vi "File Operation.vi"(8 "error in (no error)":errorcluster, 10 "Enum":T2, 11 "Cluster":T1) -> (0 "error out":errorcluster, 3 "Array":T1[][](array[typedef]))   [LabVIEW 2020]
uses:
  Controller/Product controller.ctl
  Controller/File Operation Controller.ctl
  <vilib>/Utility/config.llb/Read Key (String).vi
  <vilib>/Utility/config.llb/Read Key (I32).vi
  <vilib>/Utility/config.llb/Write Key (String).vi
  <vilib>/Utility/config.llb/NI_LVConfig.lvlib
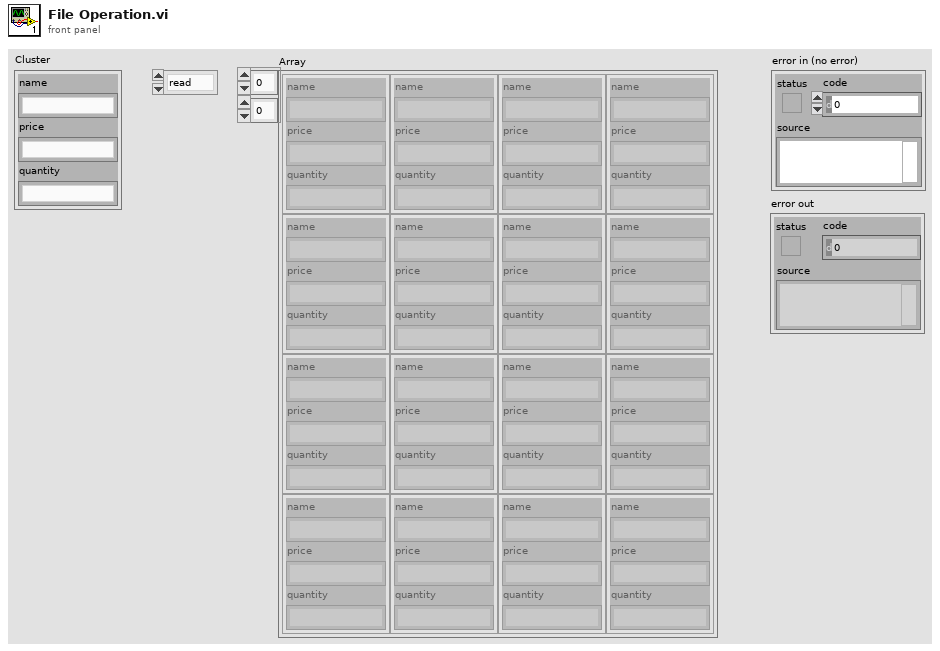
[diagram p1: front panel]
types:
  T1 = typedef "Product controller.ctl" = cluster{"name":string, "price":string, "quantity ":string}
  T2 = typedef "File Operation Controller.ctl" = enum16{"read", "write"}
  T3 = typedef "NI_LVConfig.lvlib/Config Data RefNum.ctl" = refnum<k1>
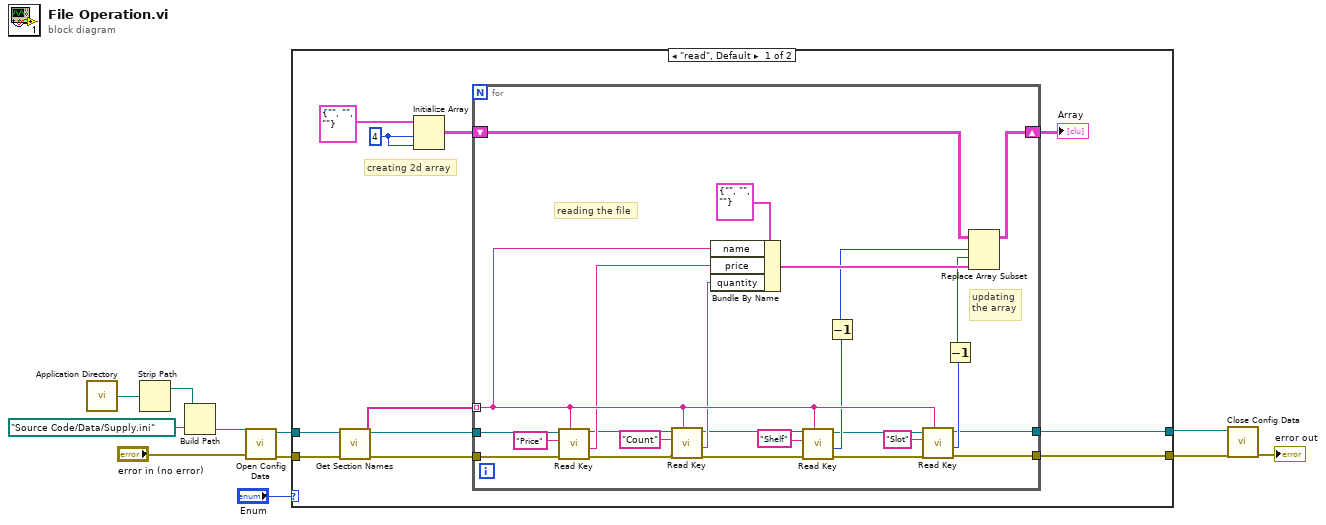
[diagram p0: block diagram]
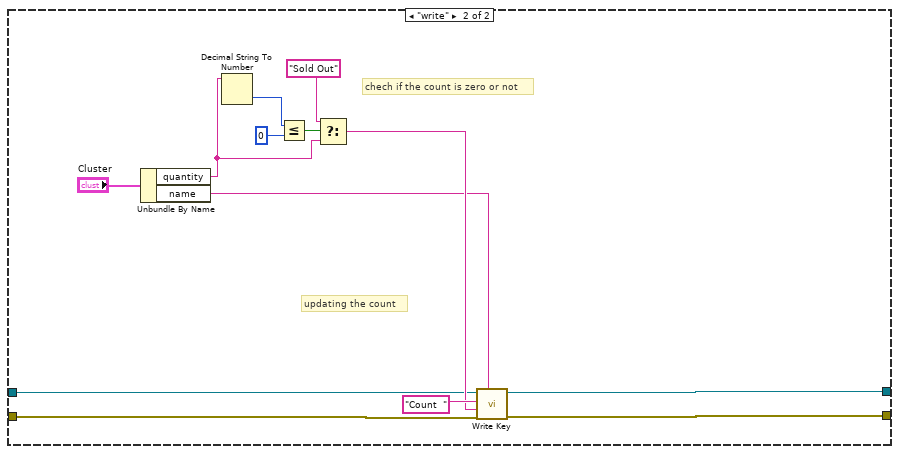
[diagram p2: hidden frame]
diagram:
  n1 = call <vilib>:"Application Directory.vi"() -> ("Application Directory"=w2:path)
  n2 = Strip Path(path=w2) -> (stripped path=w4:path)  [unwired: 1 out]
  n3 = Build Path(base path=w4, name or relative path=path "Source Code/Data/Supply.ini") -> (appended path=w1:path)
  n4 = call <vilib>:"Open Config Data.vi"("error in (no error)"="error in (no error)", "configuration file path"=w1) -> ("error out"=w10:errorcluster, "refnum"=w9:T3)  [unwired: 7 in, 1 out]
  n5 = case shown="\"read\", Default" "Enum" {
    tunnel: w10 -> [w21 w50]
    tunnel: w9 -> [w22 w51]
    tunnel: [w13 w57] -> w7
    tunnel: [w14 w58] -> w8
    frame "read", Default {
      w18 = 4 ("dimension size")
      # "creating 2d array"
      n6 = call <vilib>:"Get Section Names.vi"("error in (no error)"=w21, "refnum"=w22) -> ("error out"=w15:errorcluster, "section names"=w20:string[], "refnum out"=w12:T3)  [unwired: 7 in]
      n7 = Initialize Array(T1 {"name"="", "price"="", "quantity "=""} ("Cluster"), w18, w18) -> (w17:T1[][])
      n8 = for {
        tunnel: w20 -> [w38] mode=indexing
        shift-right: [w34] -> w16
        shift-left: w17 -> [w35]
        tunnel: w15 -> [w47]
        tunnel: [w28] -> w14
        tunnel: [w27] -> w13
        tunnel: w12 -> [w26]
        # "updating\nthe array"
        # "reading the file"
        n9 = call-poly <vilib>:"Read Key.vi"("section"=w38, "error in (no error)"=w47, "key"="Price", "refnum"=w26) -> ("error out"=w42:errorcluster, "value"=w37:string, "refnum out"=w25:T3)  [unwired: 4 in, 1 out]
        n10 = call-poly <vilib>:"Read Key.vi"("section"=w38, "error in (no error)"=w42, "key"="Count", "refnum"=w25) -> ("error out"=w41:errorcluster, "value"=w36:string, "refnum out"=w24:T3)  [unwired: 4 in, 1 out]
        n11 = Bundle By Name(cluster=T1 {"name"="", "price"="", "quantity "=""} ("Cluster"), "name"=w38, "price"=w37, "quantity"=w36) -> (w33:T1)
        n12 = call-poly <vilib>:"Read Key.vi"("section"=w38, "error in (no error)"=w41, "key"="Shelf", "refnum"=w24) -> ("error out"=w40:errorcluster, "value"=w32:i32, "refnum out"=w23:T3)  [unwired: 4 in, 1 out]
        n13 = Decrement(x=w32) -> (x-1=w30:i32)
        n14 = call-poly <vilib>:"Read Key.vi"("section"=w38, "error in (no error)"=w40, "key"="Slot", "refnum"=w23) -> ("error out"=w27:errorcluster, "value"=w31:i32, "refnum out"=w28:T3)  [unwired: 4 in, 1 out]
        n15 = Decrement(x=w31) -> (x-1=w29:i32)
        n16 = Replace Array Subset(array=w35, new element=w33, index (row)=w30, index (col)=w29) -> (w34:T1[][])
      }
      "Array" <- w16
    }
    frame "write" {
      # "updating the count"
      # "chech if the count is zero or not"
      n17 = Unbundle By Name("Cluster") -> ("quantity"=w53:string, "name"=w49:string)
      n18 = Decimal String To Number(string=w53) -> (number=w48:i32)  [unwired: 2 in, 1 out]
      n19 = Less Or Equal?(x=w48, y=0) -> (x <= y?=w55:bool)
      n20 = Select(t="Sold Out", s=w55, f=w53) -> (s? t:f=w52:string)
      n21 = call-poly <vilib>:"Write Key.vi"("section"=w49, "error in (no error)"=w50, "value"=w52, "key"="Count  ", "refnum"=w51) -> ("error out"=w57:errorcluster, "refnum out"=w58:T3)  [unwired: 4 in, 1 out]
    }
  }
  n22 = call <vilib>:"Close Config Data.vi"("error in (no error)"=w7, "refnum"=w8) -> ("error out"=→"error out":errorcluster)  [unwired: 8 in, 1 out]
